vi "Array.vi"() -> ()   [LabVIEW 2022 SP3]
panel:
  out "Array 6":dbl[](array[numeric])
  out "Numeric 2":i32
  out "Numeric":i32
  in  "Array 5":i32[](array[numeric])
  out "element":dbl
  out "size(s) 2":i32
  out "size(s)":i32[](array[numeric])
  out "Array 4":string[](array[string])
  in  "Array 3":string[](array[string])
  out "Array 2":dbl[](array[numeric])
  in  "Array":dbl[](array[numeric])
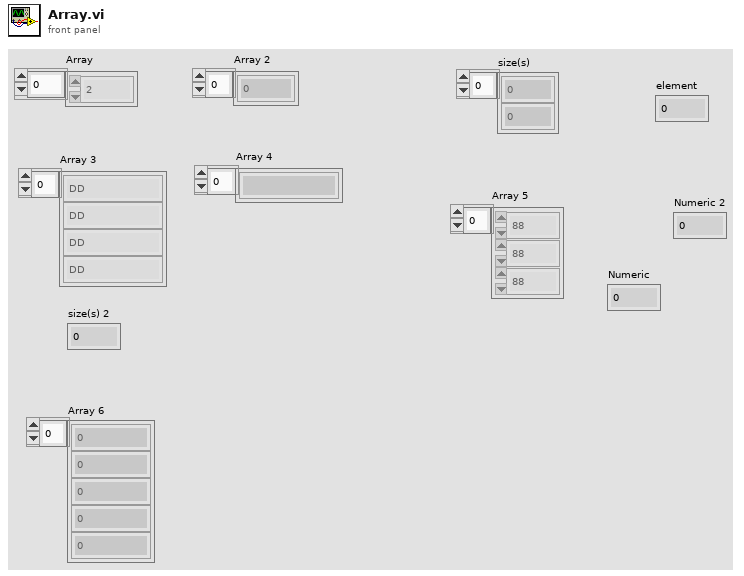
[diagram p1: front panel]
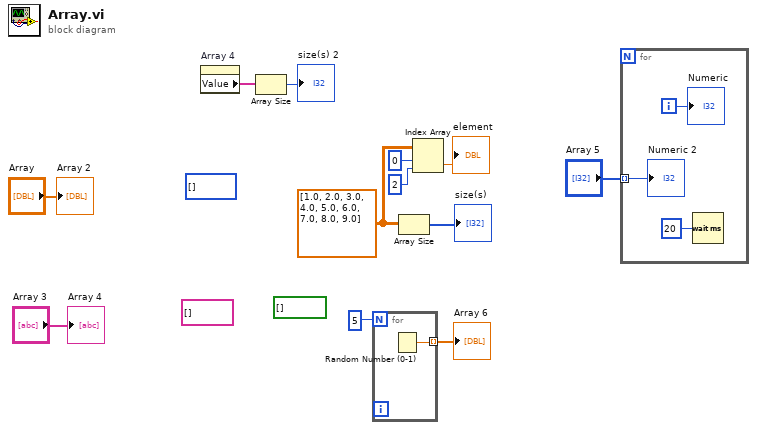
[diagram p0: block diagram]
diagram:
  (unwired) bool[] []
  (unwired) string[] []
  w7 = dbl[][] [[1.0, 2.0, 3.0], [4.0, 5.0, 6.0], [7.0, 8.0, 9.0]]
  (unwired) i32[] []
  n1 = property on="Array 4" class="Arr (strict)"() -> ("Value"=w9:string[])  [unwired: 2 in, 2 out]
  n2 = Array Size(array=w9) -> (size(s)=→"size(s) 2":i32)
  n3 = for {
    N: 5 -> [_]
    tunnel: [w13] -> w1 mode=indexing
    n4 = Random Number (0-1)() -> (number: 0 to 1=w13:dbl)
  }
  "Array 6" <- w1
  n5 = Array Size(array=w7) -> (size(s)=→"size(s)":i32[])
  n6 = Index Array(array=w7, index (row)=0, index (col)=2 ("disabled index (col)")) -> (element=→"element":dbl)
  n7 = for {
    tunnel: "Array 5" -> [w15] mode=indexing
    i -> [w16]
    n8 = Wait (ms)(milliseconds to wait=u32 20) -> ()  [unwired: 1 out]
    "Numeric" <- w16
    "Numeric 2" <- w15
  }
  "Array 2" <- "Array"
  "Array 4" <- "Array 3"
